vi "Add Line.vi"(8 "error in (no error)":errorcluster, 10 "String":string, 11 "Console Log in":refnum<class "Console Log.lvclass">) -> (0 "error out":errorcluster, 3 "Console Log out":refnum<class "Console Log.lvclass">)   [LabVIEW 2011, in "Console Log.lvclass"]
uses:
  Console Log.lvclass
  Console Log.lvclass/Console Log.ctl
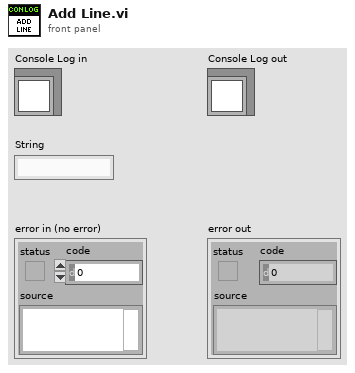
[diagram p1: front panel]
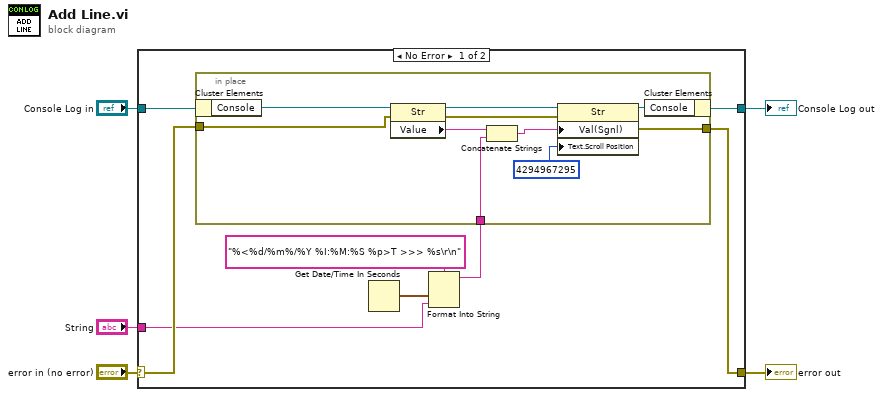
[diagram p0: block diagram]
diagram:
  n1 = case shown="No Error" "error in (no error)" {
    selector: "error in (no error)" -> [w11 w25]
    tunnel: [w10 w25] -> w4
    tunnel: [w12 w24] -> w2
    tunnel: "Console Log in" -> [w13 w24]
    tunnel: "String" -> [w8 _]
    frame No Error {
      n2 = Get Date/Time In Seconds() -> (seconds since 1Jan1904=w6:timestamp)
      n3 = Format Into String(format string="%<%d/%m%/%Y %I:%M:%S %p>T >>> %s\r\n", w6, w8) -> (resulting string=w7:string)  [unwired: 2 in, 1 out]
      n4 = in-place {
        in-place-border: w11 -> [w18]
        in-place-border: [w17] -> w10
        in-place-border: w7 -> [w15]
        n5 = in-place-cluster #1(w13) -> ("Console"=w23:refnum<vi>)
        n6 = property class="Str"(reference=w23, error in=w18) -> (reference out=w21:refnum<vi>, error out=w22:errorcluster, "Value"=w16:string)
        n7 = Concatenate Strings(w16, w15) -> (w20:string)
        n8 = property class="Str"(reference=w21, error in=w22, "Val(Sgnl)"=w20, "Text.Scroll Position"=u32 4294967295) -> (reference out=w19:refnum<vi>, error out=w17:errorcluster)
        n9 = in-place-cluster #1("Console"=w19) -> (w12:refnum<class "Console Log.lvclass">)
      }
    }
    frame Error {
    }
  }
  "error out" <- w4
  "Console Log out" <- w2
